vi "Slave.vi"() -> ()   [LabVIEW 2019]
uses:
  <vilib>/ni/Modbus Library/API/Slave/Modbus Slave.lvclass
  <vilib>/ni/Modbus Library/API/Wrapper/API Main.lvlib
panel:
  in  "Start":bool
  in  "Stop":bool
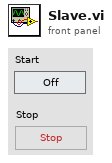
[diagram p1: front panel]
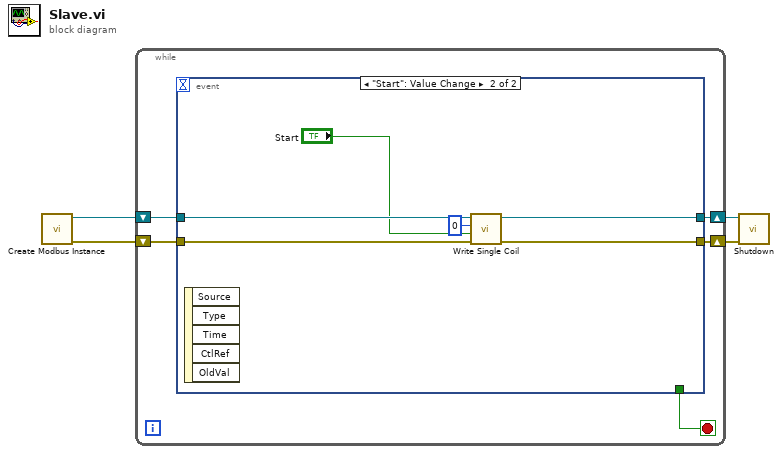
[diagram p0: block diagram]
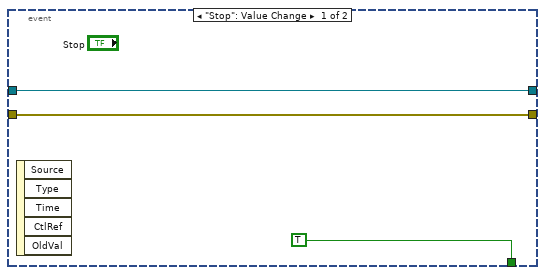
[diagram p2: hidden frame]
diagram:
  n1 = call-poly <vilib>:"Create Modbus Instance.vi"() -> ("error out"=w3:errorcluster, "TCP slave instance"=w4:refnum<class "Modbus Slave.lvclass">)  [unwired: 10 in]
  n2 = while {
    shift-right: [w6] -> w1
    shift-left: w4 -> [w9]
    shift-right: [w5] -> w2
    shift-left: w3 -> [w8]
    stop <- w7 stop-if-true
    n3 = event shown="[1] \"Start\": Value Change" {
      selector: _ -> [_ _]
      dyn-events: _ -> [_ _]
      timeout: _ -> [_ _]
      tunnel: w9 -> [w11 w18]
      tunnel: w8 -> [w10 w17]
      tunnel: [TRUE _] -> w7
      tunnel: [w11 w15] -> w6
      tunnel: [w10 w16] -> w5
      event "Stop": Value Change {
        n4 = event-data() -> ()  [unwired: 1 in, 5 out]
      }
      event "Start": Value Change {
        n5 = event-data() -> ()  [unwired: 1 in, 5 out]
        n6 = call-dynamic "Write Single Coil.vi"("error in"=w17, "coil to write"="Start", "address"=u16 0, "Modbus slave in"=w18) -> ("error out"=w16:errorcluster, "Modbus slave out"=w15:refnum<class "Modbus Slave.lvclass">)  [unwired: 6 in]
      }
    }
  }
  n7 = call-dynamic "Shutdown.vi"("error in"=w2, "Modbus slave in"=w1) -> ()  [unwired: 9 in, 1 out]
